vi "Destructor.vi"(8 "error in (no error)":errorcluster, 11 "NMR in":refnum<class "NMR.lvclass">) -> (0 "error out":errorcluster, 3 "NMR out":refnum<class "NMR.lvclass">)   [LabVIEW 2011, in "NMR.lvclass"]
uses:
  NMR.lvclass
  Communication Channel.ctl
  NMR.lvclass/NMR.ctl
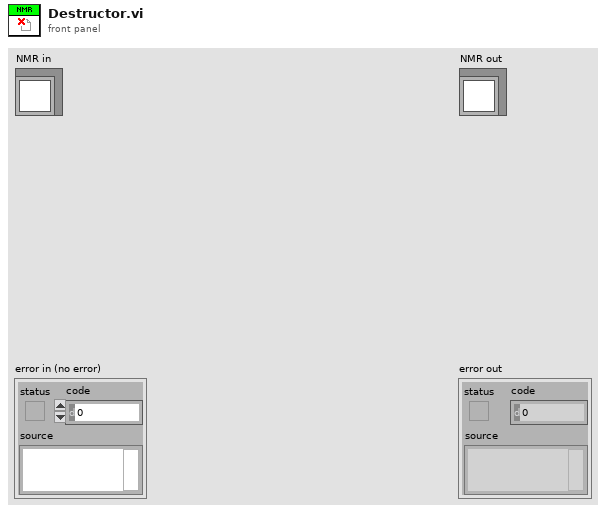
[diagram p1: front panel]
types:
  T1 = typedef "NMR.lvclass/Communication Channel.ctl" = enum16{"VISA", "DLL"}
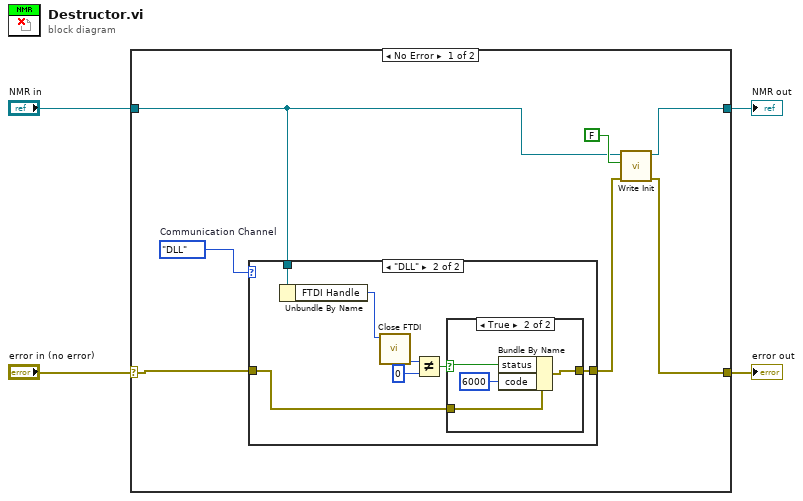
[diagram p0: block diagram]
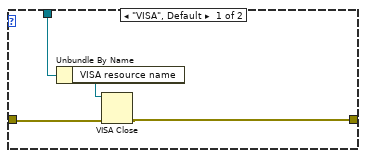
[diagram p2: hidden frame]
diagram:
  n1 = case shown="No Error" "error in (no error)" {
    selector: "error in (no error)" -> [w8 w29]
    tunnel: [w7 w29] -> w3
    tunnel: [w9 w28] -> w1
    tunnel: "NMR in" -> [w6 w28]
    frame No Error {
      w10 = Communication_Channel."DLL"  # Communication Channel
      n2 = case shown="\"DLL\"" w10 {
        tunnel: w8 -> [w12 w17]
        tunnel: [w15 w16] -> w5
        tunnel: w6 -> [w14 w22]
        frame "VISA", Default {
          n3 = Unbundle By Name(w14) -> ("VISA resource name"=w13:refnum<visa-resource-name>)
          n4 = VISA Close(VISA resource name=w13, error in (no error)=w12) -> (error out=w15:errorcluster)
        }
        frame "DLL" {
          n5 = Unbundle By Name(w22) -> ("FTDI Handle"=w21:u32)
          n6 = call "Close FTDI.vi"("FTDI Handle"=w21) -> ("FT_Status"=w20:u32)  [unwired: 10 in]
          n7 = Not Equal?(x=w20, y=u32 0) -> (x != y?=w18:bool)
          n8 = case shown="True" w18 {
            selector: w18 -> [_ w25]
            tunnel: w17 -> [w23 w27]
            tunnel: [w23 w26] -> w16
            frame False {
            }
            frame True {
              n9 = Bundle By Name(cluster=w27, "status"=w25, "code"=6000) -> (w26:errorcluster)
            }
          }
        }
      }
      n10 = call-dynamic "Write Init.vi"("error in (no error)"=w5, "Init"=FALSE, "NMR in"=w6) -> ("error out"=w7:errorcluster, "NMR out"=w9:refnum<class "NMR.lvclass">)  [unwired: 7 in]
    }
    frame Error {
    }
  }
  "error out" <- w3
  "NMR out" <- w1
